vi "List SQS Queues in Region.vi"() -> ()   [LabVIEW 2015]
doc: "Demonstrates how to list all Amazon SQS queues created by an authenticated user."
uses:
  Core/HTTP Request/Region.ctl
  Core/HTTP Request/AWS Credentials.ctl
  SQS/Queue/Queue.lvclass/Queue.ctl
  SQS/Queue/Read Name.vi
  SQS/Queue/Read URL.vi
  SQS/Queue/Queue.lvclass
  Core/HTTP Request/HTTP Request.lvclass
panel:
  in  "Region":T1
  in  "Secret Key":string
  in  "Access Key":string
  out "Queues":i32(listbox)
  # "Overview: Demonstrates how to list all Amazon SQS queues created by an authenticated user.\nRequirements: NI Cloud Toolkit for AWS and a registered Amazon AWS account\nInstructions:\n1. Specify the Access Key and Secret Key for your AWS account. You can create an account at http://aws.amazon.com.\n2. Run the VI. All the queues associated with your account should be listed in the Queues indicator."
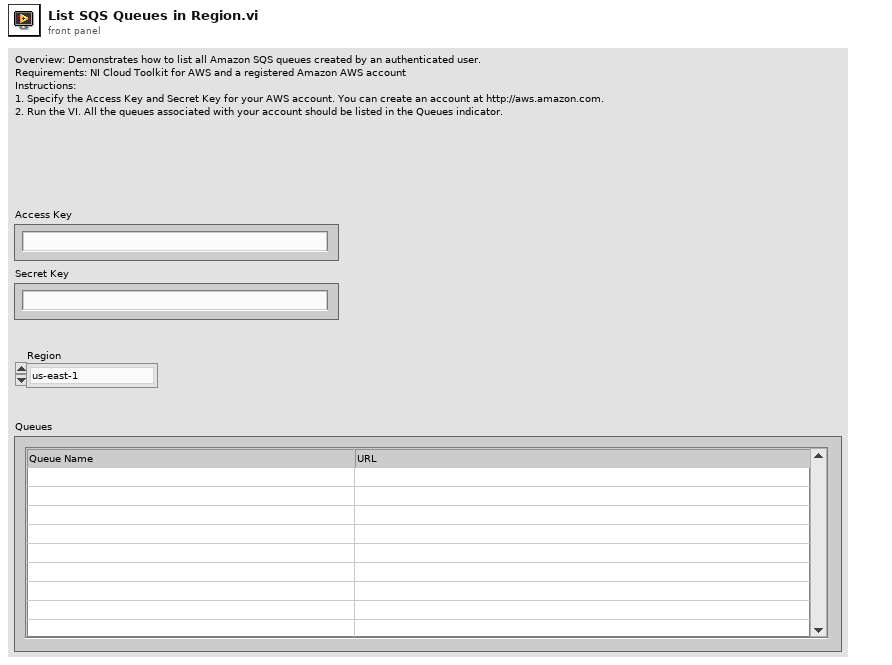
[diagram p1: front panel]
types:
  T1 = typedef "NI_AWS_Core.lvlib/HTTP Request.lvclass/Region.ctl" = enum16{"us-east-1", "us-east-2", "us-west-1", "us-west-2", "ap-northeast-1", "ap-northeast-2", "ap-southeast-1", "ap-southeast-2", "ca-central-1", "eu-central-1", "eu-west-1", "eu-west-2", "sa-east-1"}
  T2 = typedef "NI_AWS_Core.lvlib/HTTP Request.lvclass/AWS Credentials.ctl" = cluster{"Access Key":string, "Secret Key":string}
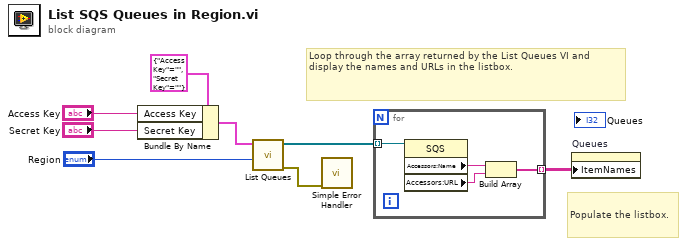
[diagram p0: block diagram]
diagram:
  # "Loop through the array returned by the List Queues VI and display the names and URLs in the listbox."
  # "Populate the listbox."
  n1 = Bundle By Name(cluster=T2 {"Access Key"="", "Secret Key"=""} ("AWS Credentials"), "Access Key"="Access Key", "Secret Key"="Secret Key") -> (w7:T2)
  n2 = call "List Queues.vi"("Region"="Region", "AWS Credentials"=w7) -> ("error out"=w1:errorcluster, "SQS Queues"=w3:refnum<class "Queue.lvclass">[])  [unwired: 8 in]
  n3 = call <vilib>:"Simple Error Handler.vi"("error in (no error)"=w1) -> ()  [unwired: 4 in, 5 out]
  n4 = for {
    tunnel: w3 -> [w12] mode=indexing
    tunnel: [w9] -> w2 mode=indexing
    n5 = property class="SQS"(reference=w12) -> ("Accessors:Name"=w11:string, "Accessors:URL"=w10:string)  [unwired: 1 in, 2 out]
    n6 = Build Array(w11, w10) -> (w9:string[])
  }
  n7 = property on="Queues" class="MCListbox (strict)"("ItemNames"=w2) -> ()  [unwired: 2 in, 2 out]
